vi "Remove_duplicate_rows.vi"() -> ()   [LabVIEW 2011]
panel:
  out "Number of Rows removed":i32
  in  "Results file":path
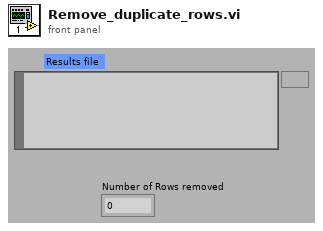
[diagram p1: front panel]
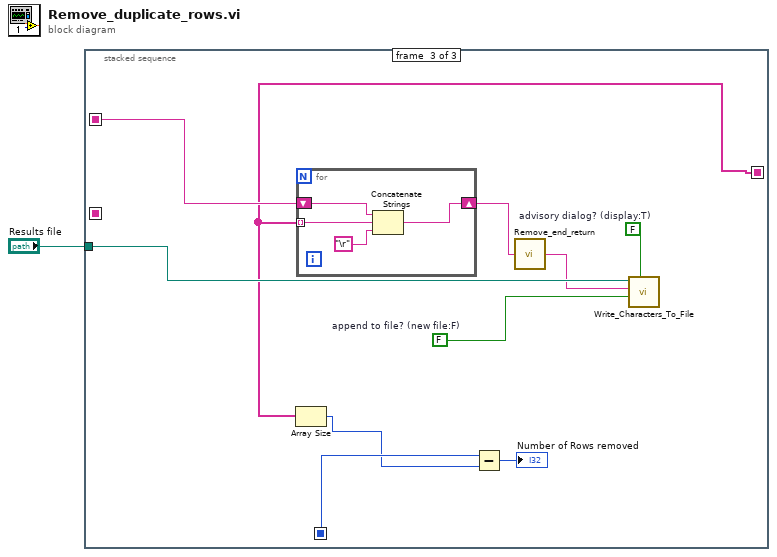
[diagram p0: block diagram]
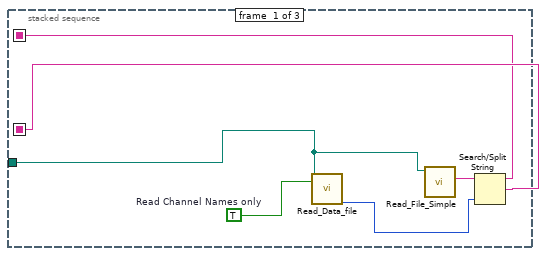
[diagram p2: hidden frame]
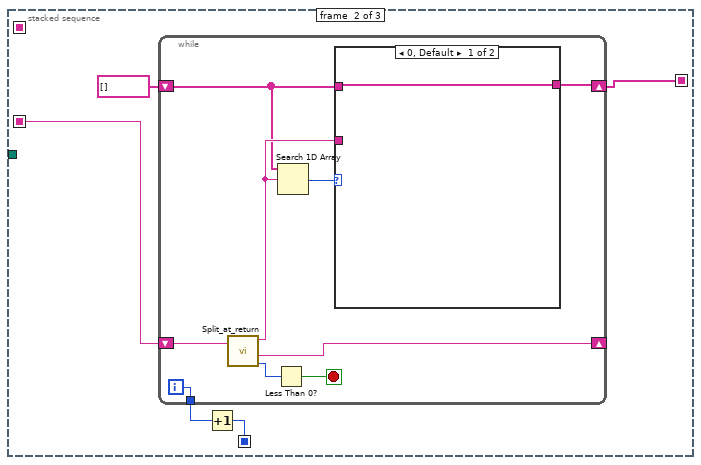
[diagram p3: hidden frame]
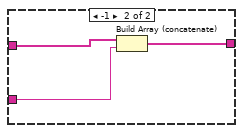
[diagram p4: hidden frame]
diagram:
  n1 = stacked-sequence {
    seq-local: [w4 _ _] -> [_ w11 _]
    seq-local: [w3 _ _] -> [_ _ w35]
    seq-local: [_ w10 _] -> [_ _ w29]
    seq-local: [_ w8 _] -> [_ _ w28]
    tunnel: "Results file" -> [w2 _ w34]
    frame #0 {
      w5 = TRUE  # Read Channel Names only
      n2 = call "Read_Data_file.vi"("Results file"=w2, "Read Channel Names only"=w5) -> ("mark after read (chars.)"=w6:i32)  [unwired: 8 in, 9 out]
      n3 = call "Read_File_Simple.vi"("Filename"=w2) -> ("string"=w7:string)  [unwired: 4 in, 5 out]
      n4 = Search/Split String(string=w7, offset (0)=w6) -> (substring before match=w3:string, match + rest of string=w4:string)  [unwired: 1 in, 1 out]
    }
    frame #1 {
      n5 = while {
        shift-right: [w20] -> _
        shift-left: w11 -> [w21]
        shift-right: [w15] -> w10
        shift-left: string[] [] -> [w14]
        tunnel: [w13] -> w9
        i -> [w13]
        stop <- w18 stop-if-true
        n6 = call "Split_at_return.vi"("String"=w21) -> ("before substring"=w16:string, "after substring"=w20:string, "offset past match"=w19:i32)  [unwired: 1 in, 1 out]
        n7 = Less Than 0?(x=w19) -> (x < 0?=w18:bool)
        n8 = Search 1D Array(1D array=w14, element=w16) -> (index of element=w17:i32)  [unwired: 1 in]
        n9 = case shown="0, Default" w17 {
          tunnel: w14 -> [w22 w25]
          tunnel: w16 -> [_ w24]
          tunnel: [w22 w23] -> w15
          frame 0, Default {
          }
          frame -1 {
            n10 = Build Array (concatenate)(w25, w24) -> (w23:string[])
          }
        }
      }
      n11 = Increment(x=w9) -> (x+1=w8:i32)
    }
    frame #2 {
      w32 = FALSE  # append to file? (new file:F)
      w33 = FALSE  # advisory dialog? (display:T)
      n12 = Array Size(array=w29) -> (size(s)=w27:i32)
      n13 = for {
        shift-right: [w36] -> w31
        shift-left: w35 -> [w37]
        tunnel: w29 -> [w38] mode=indexing
        n14 = Concatenate Strings(w37, w38, "\r") -> (w36:string)
      }
      n15 = Subtract(x=w28, y=w27) -> (x-y=→"Number of Rows removed":i32)
      n16 = call "Remove_end_return.vi"("Input string"=w31) -> ("Output string"=w30:string)
      n17 = call "Write_Characters_To_File.vi"("file path (dialog if empty)"=w34, "advisory dialog? (display:T)"=w33, "character string"=w30, "append to file? (new file:F)"=w32) -> ()  [unwired: 4 in, 1 out]
    }
  }
